vi "Insert New Test Data.vi"(8 "error in (no error)":errorcluster, 10 "Test Data":T1, 11 "Session Handle in":T4) -> (0 "error out":errorcluster, 3 "Session Handle out":T4)   [LabVIEW 2018, in "TestDataMgr.lvclass"]
uses:
  TestDataMgr.lvclass
  Typedefs/Session Handle.ctl
  Typedefs/Test Data All.ctl
  Typedefs/Test Limits.ctl
  Typedefs/Test Raw Data.ctl
  TestDataMgr.lvclass/TestDataMgr.ctl
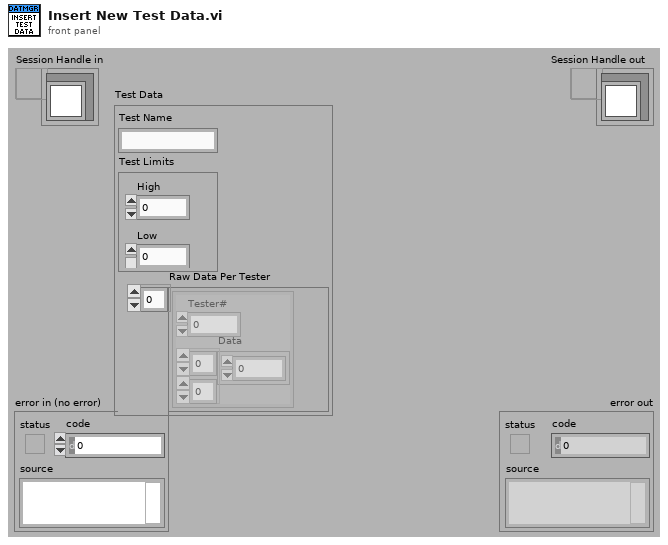
[diagram p1: front panel]
types:
  T1 = typedef "TestDataMgr.lvclass/Test Data All.ctl" = cluster{"Test Name":string, "Test Limits":T2, "Raw Data Per Tester":T3[]}
  T2 = typedef "TestDataMgr.lvclass/Test Limits.ctl" = cluster{"High":dbl, "Low":dbl}
  T3 = typedef "TestDataMgr.lvclass/Test Raw Data.ctl" = cluster{"Data":dbl[][], "Tester#":u8}
  T4 = typedef "TestDataMgr.lvclass/Session Handle.ctl" = refnum<data-value>
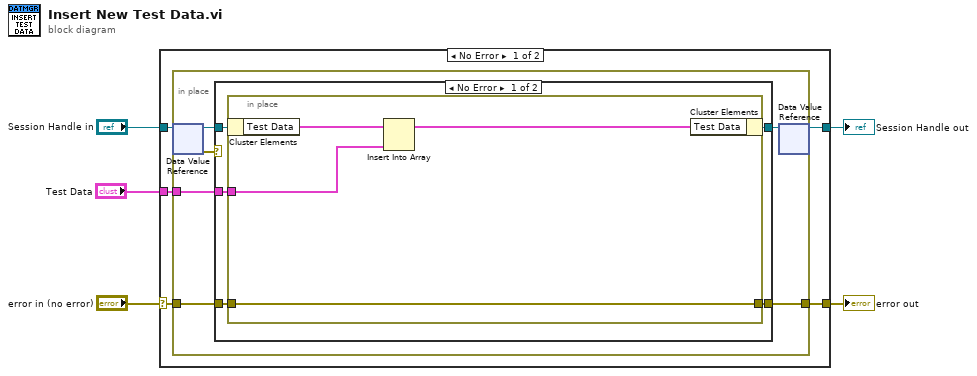
[diagram p0: block diagram]
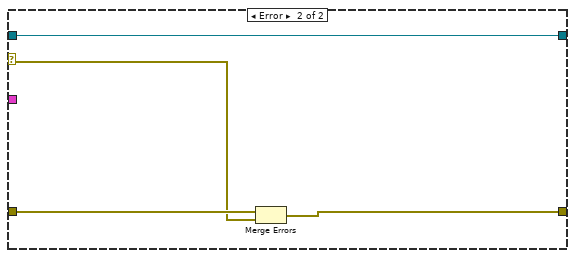
[diagram p2: hidden frame]
diagram:
  n1 = case shown="No Error" "error in (no error)" {
    selector: "error in (no error)" -> [w8 w30]
    tunnel: "Session Handle in" -> [w10 w31]
    tunnel: [w9 w31] -> w4
    tunnel: [w7 w30] -> w3
    tunnel: "Test Data" -> [w6 _]
    frame No Error {
      n2 = in-place {
        in-place-border: w8 -> [w12]
        in-place-border: [w15] -> w7
        in-place-border: w6 -> [w11]
        n3 = in-place-dvr #1(w10) -> (w16:refnum<class "TestDataMgr.lvclass">, w13:errorcluster)
        n4 = case shown="No Error" w13 {
          selector: w13 -> [_ w28]
          tunnel: w16 -> [w21 w26]
          tunnel: [w20 w27] -> w15
          tunnel: [w19 w26] -> w14
          tunnel: w12 -> [w18 w29]
          tunnel: w11 -> [w17 _]
          frame No Error {
            n5 = in-place {
              in-place-border: [w25] -> w20
              in-place-border: w18 -> [w25]
              in-place-border: w17 -> [w23]
              n6 = in-place-cluster #2(w21) -> ("Test Data"=w24:T1[])
              n7 = Insert Into Array(array=w24, new element=w23) -> (w22:T1[])  [unwired: 1 in]
              n8 = in-place-cluster #2("Test Data"=w22) -> (w19:refnum<class "TestDataMgr.lvclass">)
            }
          }
          frame Error {
            n9 = Merge Errors(w29, w28) -> (w27:errorcluster)
          }
        }
        n10 = in-place-dvr #1(w14) -> (w9:T4)  [unwired: 1 out]
      }
    }
    frame Error {
    }
  }
  "Session Handle out" <- w4
  "error out" <- w3
